vi "RemoteForKeyboard.vi"() -> ()   [LabVIEW 2020]
uses:
  <vilib>/CISH Robotics/L4VMX TitanQuad/Motor ID.ctl
  <vilib>/CISH Robotics/L4VMX VMXpi/Type Def/VMX Channel Index.ctl
  <vilib>/ReMiSYS Technology/RemoteToolkit/Receiver/Receiver.lvclass
  <vilib>/CISH Robotics/L4VMX VMXpi/L4VMX.lvlib
  <vilib>/CISH Robotics/L4VMX VMXpi/Digital Input/Digital Input.lvclass
  <vilib>/CISH Robotics/L4VMX TitanQuad/TitanQuad.lvclass
panel:
  out "XY Speed":cluster{"X":i8, "Y":i8}
  out "Stop0":bool
  out "Error Out":errorcluster
  in  "Stop":bool
  out "Received?":bool
  # "61 * 16"
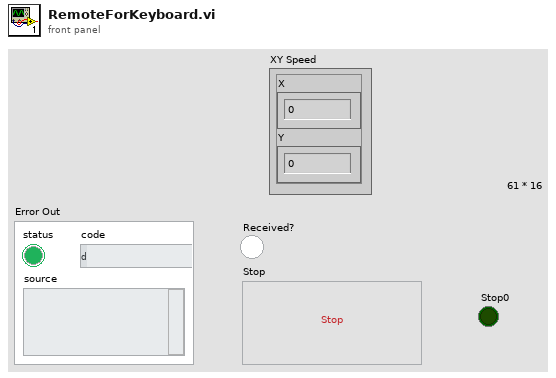
[diagram p1: front panel]
types:
  T1 = typedef "TitanQuad.lvlib/TitanQuad.lvclass/Motor ID.ctl" = enum16{"M0", "M1", "M2", "M3"}
  T2 = typedef "L4VMX.lvlib/VMX Channel Index.ctl" = enum16{"0", "1", "2", "3", "4", "5", "6", "7", "8", "9", "10", "11", "12", "13", "14", "15", "16", "17", "18", "19", "20", "21", "22", "23", "24", "25", "26", "27", "28", "29", "30", "31", "32", "33"}
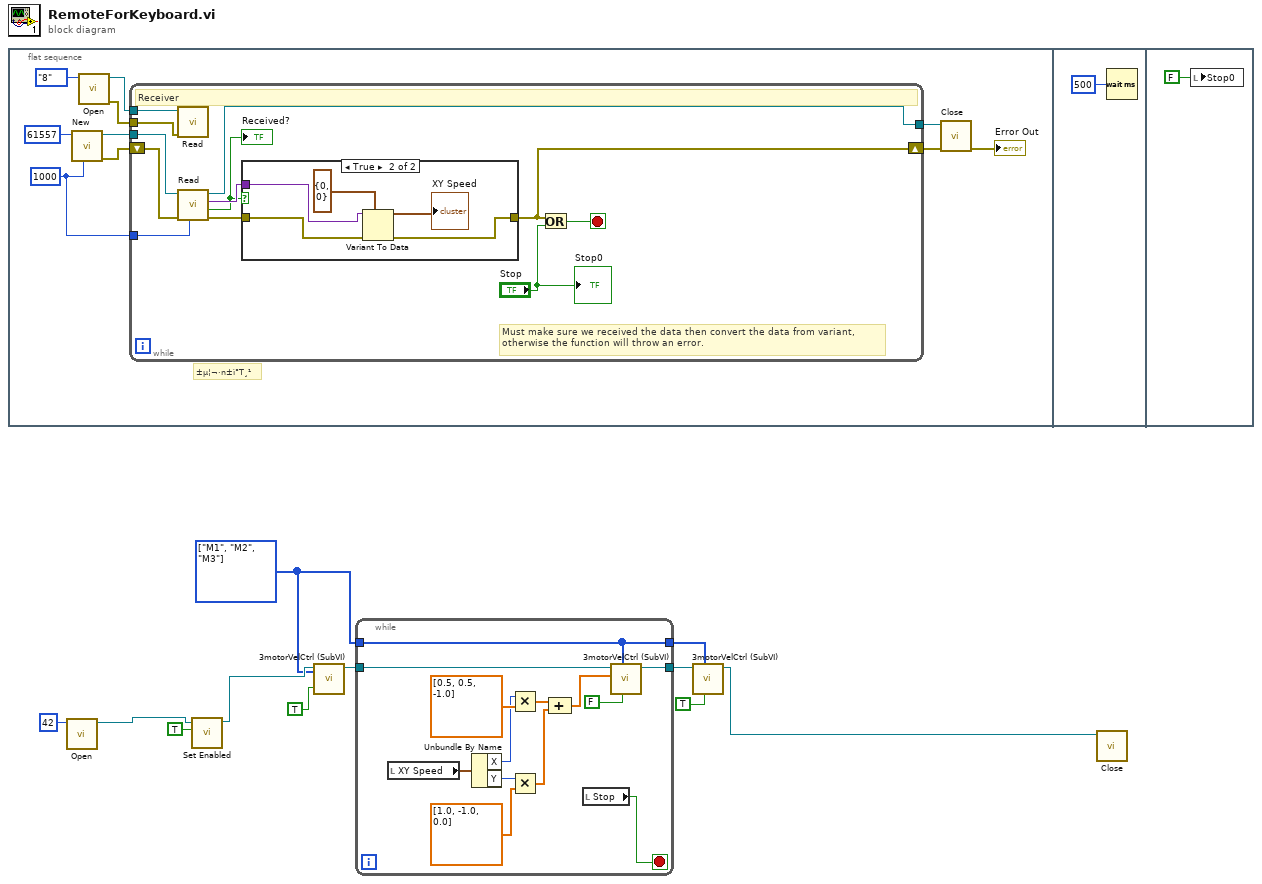
[diagram p0: block diagram]
diagram:
  w2 = T1[] [enum."M1", enum."M2", enum."M3"] items=["M0", "M1", "M2", "M3"] ("motorPort [M0, M1, M2]")
  n1 = flat-sequence {
    frame #0 {
      w17 = 1000 ("Timeout ms (25000)")
      # "±µ¦¬·n±ì°T¸¹"
      n2 = call <vilib>:"New.vi"("Timeout ms (25000)"=w17, "Port (61557)"=u16 61557) -> ("Error Out"=w21:errorcluster, "Receiver Ref."=w20:refnum<class "Receiver.lvclass">)  [unwired: 8 in]
      n3 = call <vilib>:"Open.vi"("VMX Channel Index"=VMX_Channel_Index."8") -> ("Error Out"=w12:errorcluster, "Digital Input Object"=w13:refnum<class "Digital Input.lvclass">)  [unwired: 9 in]
      n4 = while {
        shift-right: [w26] -> w19
        shift-left: w21 -> [w33]
        tunnel: w20 -> [w32]
        tunnel: [w31] -> w18
        tunnel: w17 -> [w30]
        tunnel: w13 -> [w24]
        tunnel: w12 -> [w23]
        stop <- w29 stop-if-true
        # "Must make sure we received the data then convert the data from variant,\notherwise the function will throw an error."
        # "Receiver"
        n5 = call <vilib>:"Read.vi"("Error In"=w23, "Digital Input Object"=w24) -> ()  [unwired: 7 in, 3 out]
        n6 = call <vilib>:"Read.vi"("Timeout ms (1000)"=w30, "Error In"=w33, "Receiver Ref."=w32) -> ("Error Out"=w28:errorcluster, "Received?"=w25:bool, "Value"=w27:variant, "Receiver Ref."=w31:refnum<class "Receiver.lvclass">)  [unwired: 5 in]
        "Received?" <- w25
        n7 = case shown="True" w25 {
          tunnel: w28 -> [w34 w39]
          tunnel: w27 -> [_ w38]
          tunnel: [w34 w37] -> w26
          frame False {
          }
          frame True {
            n8 = Variant To Data(error in=w39, type=cluster{"Output":i8, "Output":i8} {"Output"=0, "Output"=0} ("XY Speed"), Variant=w38) -> (data=→"XY Speed":cluster{"Output":i8, "Output":i8}, error out=w37:errorcluster)
          }
        }
        n9 = Or(x=w26, y="Stop") -> (x .or. y?=w29:bool)
        "Stop0" <- "Stop"
      }
      n10 = call <vilib>:"Close.vi"("Error In"=w19, "Receiver Ref."=w18) -> ("Error Out"=→"Error Out":errorcluster)  [unwired: 9 in]
    }
    frame #1 {
      n11 = Wait (ms)(milliseconds to wait=u32 500) -> ()  [unwired: 1 out]
    }
    frame #2 {
      n12 = local write "Stop0"(FALSE ("Stop")) -> ()
    }
  }
  n13 = call <vilib>:"Open.vi"("Titan ID (42)"=u8 42) -> ("TitanQuad Object"=w11:refnum<class "TitanQuad.lvclass">)  [unwired: 9 in, 1 out]
  n14 = call <vilib>:"Set Enabled.vi"("Enable"=TRUE, "TitanQuad Object"=w11) -> ("TitanQuad Object"=w8:refnum<class "TitanQuad.lvclass">)  [unwired: 8 in, 1 out]
  n15 = call "3motorVelCtrl (SubVI).vi"("reset Encoder"=TRUE, "motorPort [M0, M1, M2]"=w2, "TitanQuad in"=w8) -> ("TitanQuad out"=w7:refnum<class "TitanQuad.lvclass">)  [unwired: 6 in, 2 out]
  n16 = while {
    tunnel: w7 -> [w47]
    tunnel: [w46] -> w5
    tunnel: [w43] -> w3
    tunnel: w2 -> [w43]
    stop <- w42 stop-if-true
    n17 = local read "XY Speed"() -> (w54:cluster{"X":i8, "Y":i8})
    n18 = Unbundle By Name(w54) -> ("X"=w49:i8, "Y"=w48:i8)
    n19 = Multiply(x=w49, y=dbl[] [0.5, 0.5, -1.0]) -> (x*y=w51:dbl[])
    n20 = Multiply(x=w48, y=dbl[] [1.0, -1.0, 0.0]) -> (x*y=w50:dbl[])
    n21 = Compound Arithmetic op=ADD(w51, w50) -> (w45:dbl[])
    n22 = local read "Stop"() -> (w42:bool)
    n23 = call "3motorVelCtrl (SubVI).vi"("reset Encoder"=FALSE, "motorPort [M0, M1, M2]"=w43, "motorSpeed [M0, M1, M2] (deg/s)"=w45, "TitanQuad in"=w47) -> ("TitanQuad out"=w46:refnum<class "TitanQuad.lvclass">)  [unwired: 5 in, 2 out]
  }
  n24 = call "3motorVelCtrl (SubVI).vi"("reset Encoder"=TRUE, "motorPort [M0, M1, M2]"=w3, "TitanQuad in"=w5) -> ("TitanQuad out"=w4:refnum<class "TitanQuad.lvclass">)  [unwired: 6 in, 2 out]
  n25 = call <vilib>:"Close.vi"("TitanQuad Object"=w4) -> ()  [unwired: 10 in, 1 out]
